vi "Dequeue.vi"(0 "queue in":refnum<queue>, 1 "Dequeue Type":T1, 11 "error in (no error)":errorcluster) -> (4 "queue out":refnum<queue>, 6 "Message":string, 8 "Message Data":variant, 10 "MyPluginsClass":refnum<class "MyPluginsBase.lvclass">, 15 "error out":errorcluster)   [LabVIEW 2018, in "MyPlugins.lvlib"]
doc: "Dequeues a message and message data from a queue based on the queue name."
uses:
  MyPlugins.lvlib
  DequeueTypes.ctl
  MyPluggableModule/PublicAPI/Arguments/Messages/clMessage.ctl
  MyPluginBaseClass/MyPluginsBase.lvclass
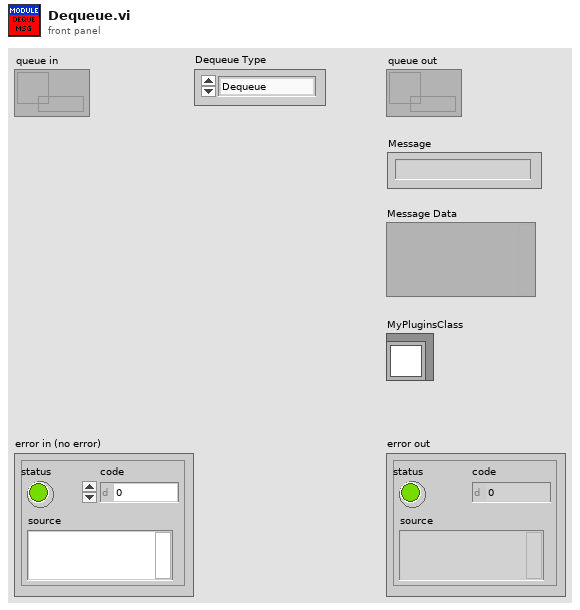
[diagram p1: front panel]
types:
  T1 = typedef "MyPlugins.lvlib/DequeueTypes.ctl" = enum16{"Dequeue", "Preview Queue"}
  T2 = typedef "MyPlugins.lvlib/clMessage.ctl" = cluster{"Message":string, "Message Data":variant, "MyPluginsClass":refnum<class "MyPluginsBase.lvclass">}
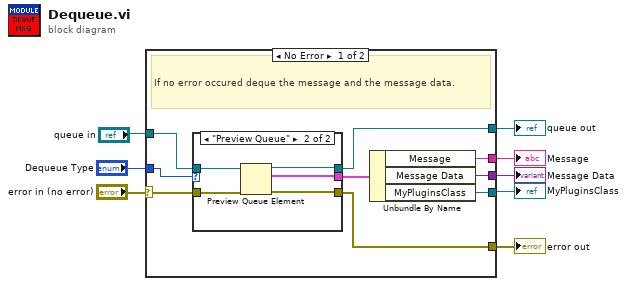
[diagram p0: block diagram]
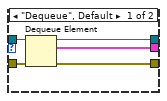
[diagram p2: hidden frame]
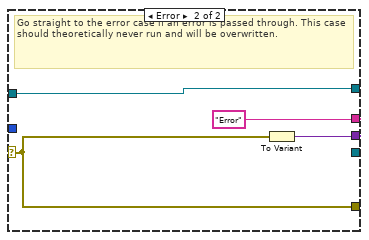
[diagram p3: hidden frame]
diagram:
  n1 = case shown="No Error" "error in (no error)" {
    selector: "error in (no error)" -> [w14 w30]
    tunnel: "queue in" -> [w12 w28]
    tunnel: [w16 w30] -> w7
    tunnel: [w15 "Error" ("Message")] -> w6
    tunnel: [w13 w29] -> w5
    tunnel: [w11 w28] -> w3
    tunnel: [w10 _] -> w2
    tunnel: "Dequeue Type" -> [w9 _]
    frame No Error {
      # "If no error occured deque the message and the message data."
      n2 = case shown="\"Preview Queue\"" w9 {
        tunnel: [w22 w23] -> w17
        tunnel: [w21 w24] -> w16
        tunnel: w14 -> [w20 w27]
        tunnel: w12 -> [w19 w26]
        tunnel: [w18 w25] -> w11
        frame "Dequeue", Default {
          n3 = Dequeue Element(queue=w19, error in (no error)=w20) -> (queue out=w18:refnum<queue>, element=w22:T2, error out=w21:errorcluster)  [unwired: 1 in, 1 out]
        }
        frame "Preview Queue" {
          n4 = Preview Queue Element(queue=w26, error in (no error)=w27) -> (queue out=w25:refnum<queue>, element=w23:T2, error out=w24:errorcluster)  [unwired: 1 in, 1 out]
        }
      }
      n5 = Unbundle By Name(w17) -> ("Message"=w15:string, "Message Data"=w13:variant, "MyPluginsClass"=w10:refnum<class "MyPluginsBase.lvclass">)
    }
    frame Error {
      # "Go straight to the error case if an error is passed through. This case should theoretically never run and will be overwritten."
      n6 = To Variant(anything=w30) -> (Variant=w29:variant)
    }
  }
  "error out" <- w7
  "Message" <- w6
  "Message Data" <- w5
  "queue out" <- w3
  "MyPluginsClass" <- w2
